vi "invalidate bad data timestamps.vi"(4 "scans per write":u16=20, 6 "output type order":T1[](array[typedef]), 7 "sample counter":i32, 8 "error in":errorcluster, 10 "cache allocation in":T2, 11 "tdms file in":refnum<k34>) -> (0 "error out":errorcluster, 2 "cache allocation out":T2, 3 "tdms file out":refnum<k34>)   [LabVIEW 2013, in "TDMS datalogger runtime.lvclass"]
uses:
  TDMS datalogger runtime.lvclass
  data cache.ctl
  <vilib>/NI/Tag Bus/tag/Data Type.ctl
  <vilib>/NI/Tag Bus/tag/tag descriptor.lvclass
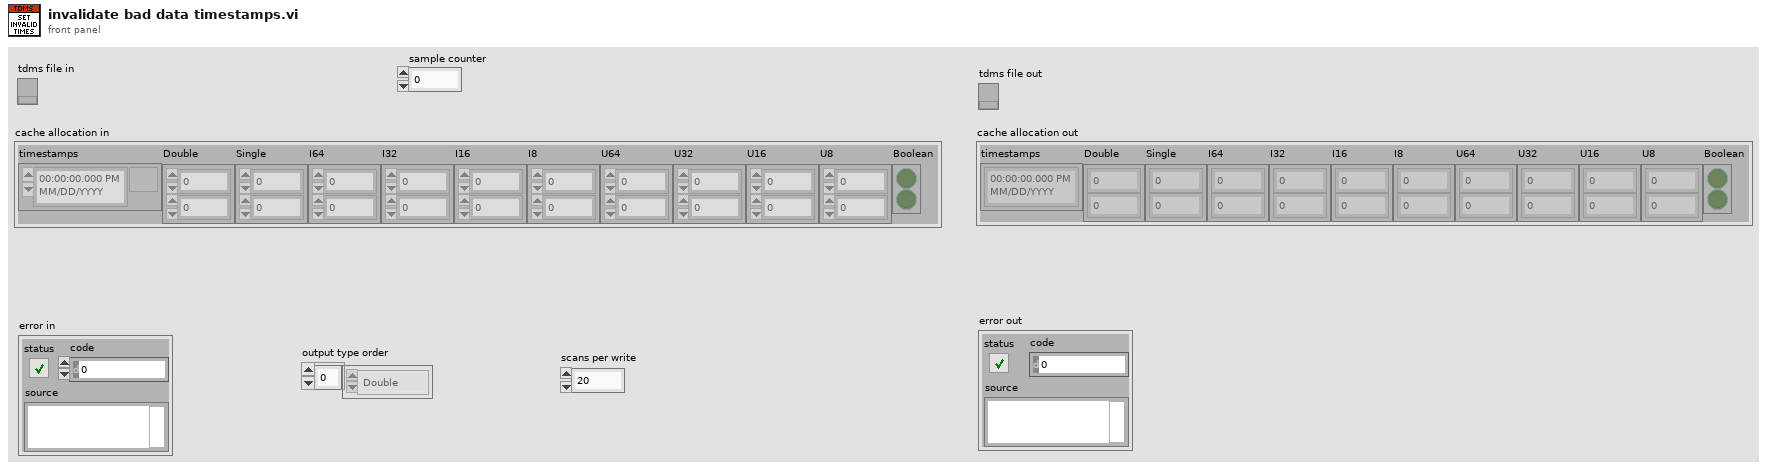
[diagram p1: front panel]
types:
  T1 = typedef "tag bus.lvlib/tag descriptor.lvclass/Data Type.ctl" = enum16{"Double", "Single", "I64", "I32", "I16", "I8", "U64", "U32", "U16", "U8", "Boolean", "String", "Array of Double", "Array of Single", "Array of I64", "Array of I32", "Array of I16", "Array of I8", "Array of U64", "Array of U32", "Array of U16", "Array of U8", "Array of Boolean", "Array of String"}
  T2 = typedef "TDMS datalogger runtime.lvclass/data cache.ctl" = cluster{"timestamps":timestamp[], "Double":dbl[][], "Single":sgl[][], "I64":i64[][], "I32":i32[][], "I16":i16[][], "I8":i8[][], "U64":u64[][], "U32":u32[][], "U16":u16[][], "U8":u8[][], "Boolean":bool[][]}
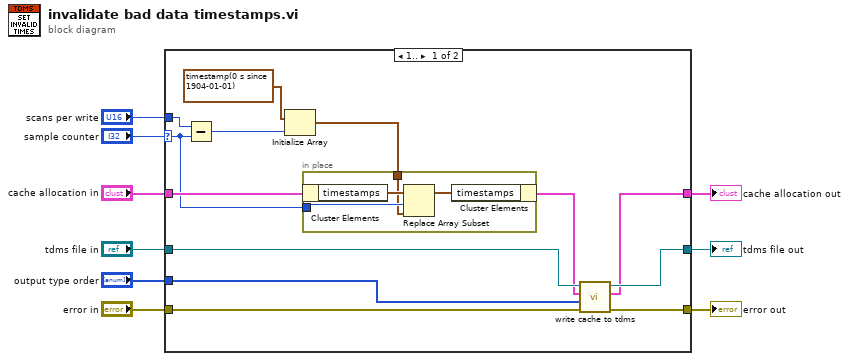
[diagram p0: block diagram]
diagram:
  n1 = case shown="1.." "sample counter" {
    selector: "sample counter" -> [w20 _]
    tunnel: "cache allocation in" -> [w21 w27]
    tunnel: "error in" -> [w16 w28]
    tunnel: "output type order" -> [w10 _]
    tunnel: "tdms file in" -> [w15 w29]
    tunnel: [w14 w29] -> w4
    tunnel: [w13 w28] -> w3
    tunnel: [w11 w27] -> w2
    tunnel: "scans per write" -> [w22 _]
    frame 1.. {
      n2 = Subtract(x=w22, y=w20) -> (x-y=w19:i32)
      n3 = Initialize Array(timestamp(0 s since 1904-01-01), w19) -> (w17:timestamp[])
      n4 = in-place {
        in-place-border: w20 -> [w24]
        in-place-border: w17 -> [w23]
        n5 = in-place-cluster #1(w21) -> ("timestamps"=w26:timestamp[])
        n6 = Replace Array Subset(array=w26, new element=w23, index=w24) -> (w25:timestamp[])
        n7 = in-place-cluster #1("timestamps"=w25) -> (w12:T2)
      }
      n8 = call "write cache to tdms.vi"("error in"=w16, "output type order"=w10, "cache in"=w12, "tdms file in"=w15) -> ("error out"=w13:errorcluster, "cache out"=w11:T2, "tdms file out"=w14:refnum<k34>)  [unwired: 5 in]
    }
    frame 0, Default {
    }
  }
  "cache allocation out" <- w2
  "tdms file out" <- w4
  "error out" <- w3
